vi "Check Path Name.vi"(9 "Error Message in":string, 10 "Valid in":bool, 11 "New Project Path":path) -> (1 "Error Message out":string, 2 "Valid out":bool)   [LabVIEW 2021, in "CIF_Plugin_Generator.lvclass"]
uses:
  CIF_Plugin_Generator.lvclass
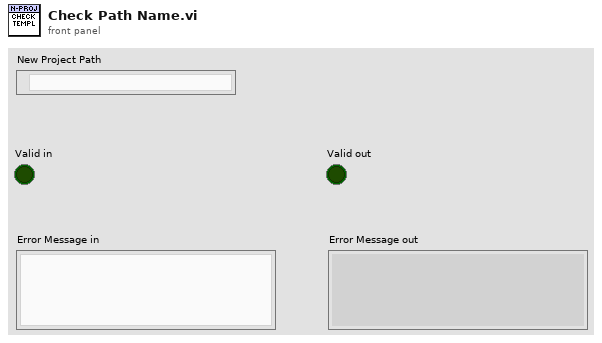
[diagram p1: front panel]
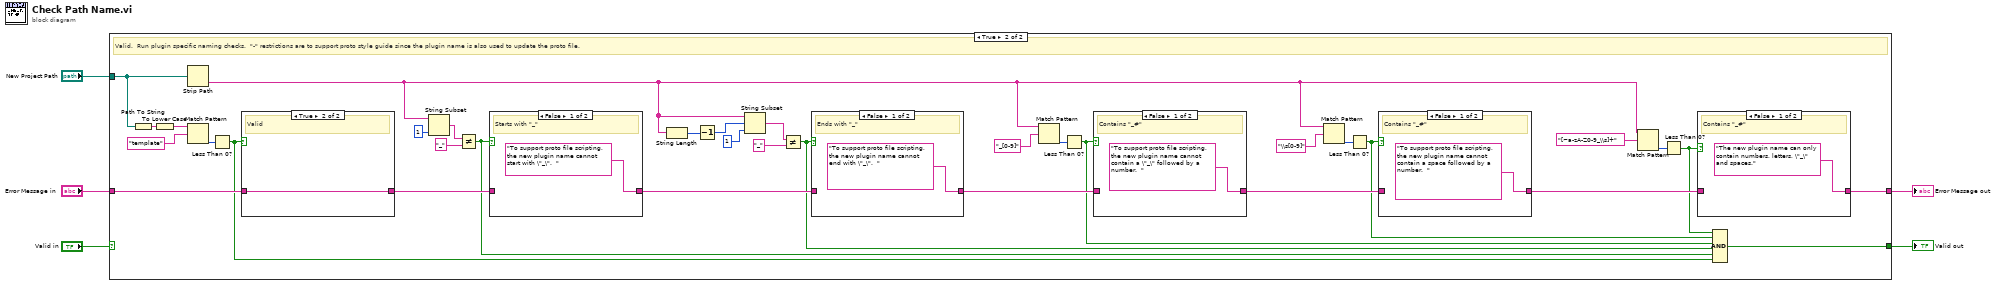
[diagram p0: block diagram]
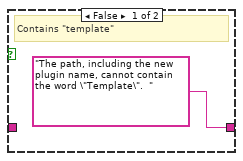
[diagram p8: hidden frame]
diagram:
  n1 = case shown="True" "Valid in" {
    selector: "Valid in" -> [w6 _]
    tunnel: "New Project Path" -> [_ w31]
    tunnel: "Error Message in" -> [w7 w30]
    tunnel: [w7 w15] -> w3
    tunnel: [w6 w18] -> w1
    frame False {
      # "Invalid name"
    }
    frame True {
      # "Valid.  Run plugin specific naming checks.  \"-\" restrictions are to support proto style guide since the plugin name is also used to update the proto file."
      n2 = Path To String(path=w31) -> (string=w35:string)
      n3 = To Lower Case(string=w35) -> (all lower case string=w34:string)
      n4 = Strip Path(path=w31) -> (name=w10:string)  [unwired: 1 out]
      n5 = Match Pattern(string=w34, regular expression="template") -> (offset past match=w32:i32)  [unwired: 1 in, 3 out]
      n6 = Less Than 0?(x=w32) -> (x < 0?=w19:bool)
      n7 = case shown="True" w19 {
        tunnel: w30 -> [_ w53]
        tunnel: ["The path, including the new plugin name, cannot contain the word \"Template\".  " ("Contains Template") w53] -> w29
        frame False {
          # "Contains \"template\""
        }
        frame True {
          # "Valid"
        }
      }
      n8 = String Subset(string=w10, length (rest)=1 ("length (rest)")) -> (substring=w40:string)  [unwired: 1 in]
      n9 = Not Equal?(x=w40, y="_") -> (x != y?=w20:bool)
      n10 = case shown="False" w20 {
        tunnel: w29 -> [_ w51]
        tunnel: ["To support proto file scripting, the new plugin name cannot start with \"_\".  " ("Contains Template") w51] -> w25
        frame False {
          # "Starts with \"_\""
        }
        frame True {
          # "Valid"
        }
      }
      n11 = String Length(string=w10) -> (length=w41:i32)
      n12 = Decrement(x=w41) -> (x-1=w37:i32)
      n13 = String Subset(string=w10, offset (0)=w37, length (rest)=1 ("length (rest)")) -> (substring=w39:string)
      n14 = Not Equal?(x=w39, y="_") -> (x != y?=w21:bool)
      n15 = case shown="False" w21 {
        tunnel: w25 -> [_ w49]
        tunnel: ["To support proto file scripting, the new plugin name cannot end with \"_\".  " ("Contains Template") w49] -> w24
        frame False {
          # "Ends with \"_\""
        }
        frame True {
          # "Valid"
        }
      }
      n16 = Match Pattern(string=w10, regular expression="_[0-9]") -> (offset past match=w36:i32)  [unwired: 1 in, 3 out]
      n17 = Less Than 0?(x=w36) -> (x < 0?=w22:bool)
      n18 = case shown="False" w22 {
        tunnel: w24 -> [_ w47]
        tunnel: ["To support proto file scripting, the new plugin name cannot contain a \"_\" followed by a number.  " ("Contains Template") w47] -> w12
        frame False {
          # "Contains \"_#\""
        }
        frame True {
          # "Valid"
        }
      }
      n19 = Match Pattern(string=w10, regular expression="\\s[0-9]") -> (offset past match=w13:i32)  [unwired: 1 in, 3 out]
      n20 = Less Than 0?(x=w13) -> (x < 0?=w8:bool)
      n21 = case shown="False" w8 {
        tunnel: w12 -> [_ w43]
        tunnel: ["To support proto file scripting, the new plugin name cannot contain a space followed by a number.  " ("Contains Template") w43] -> w11
        frame False {
          # "Contains \"_#\""
        }
        frame True {
          # "Valid"
        }
      }
      n22 = Match Pattern(string=w10, regular expression="[~a-zA-Z0-9_\\s]+") -> (offset past match=w16:i32)  [unwired: 1 in, 3 out]
      n23 = Less Than 0?(x=w16) -> (x < 0?=w9:bool)
      n24 = case shown="False" w9 {
        tunnel: w11 -> [_ w45]
        tunnel: ["The new plugin name can only contain numbers, letters, \"_\" and spaces." ("Contains Template") w45] -> w15
        frame False {
          # "Contains \"_#\""
        }
        frame True {
          # "Valid"
        }
      }
      n25 = Compound Arithmetic op=AND(w9, w8, w22, w21, w20, w19) -> (w18:bool)
    }
  }
  "Error Message out" <- w3
  "Valid out" <- w1
